vi "Dbl2Int.vi"(11 "AO_converted [V]":dbl) -> (3 "AO_raw":i16)   [LabVIEW 2020, in "FPGA_IO.lvlib"]
doc: "Convert floating point (DBL) values into 12-bit AI integer values."
uses:
  FPGA_IO.lvlib
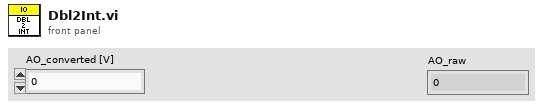
[diagram p1: front panel]
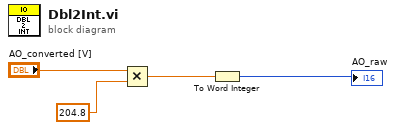
[diagram p0: block diagram]
diagram:
  n1 = Multiply(x="AO_converted [V]", y=204.8) -> (x*y=w2:dbl)
  n2 = To Word Integer(number=w2) -> (16bit integer=→"AO_raw":i16)
